vi "0 - 19 NUMBER TO STRING(SubVI).vi"(1 "A":i32) -> (0 "element":string)   [LabVIEW 2019]
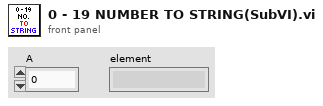
[diagram p1: front panel]
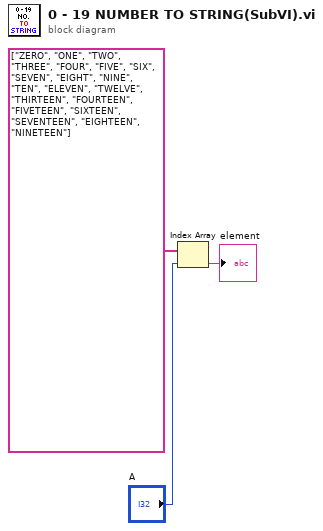
[diagram p0: block diagram]
diagram:
  n1 = Index Array(array=string[] ["ZERO", "ONE", "TWO", "THREE", "FOUR", "FIVE", "SIX", "SEVEN", "EIGHT", "NINE", "TEN", "ELEVEN", "TWELVE", "THIRTEEN", "FOURTEEN", "FIVETEEN", "SIXTEEN", "SEVENTEEN", "EIGHTEEN", "NINETEEN"], index="A") -> (element=→"element":string)
